vi "1D Look-Up Table.vi"   [LabVIEW 2017, in "NI_AdvCtrl_nonlinear.lvlib"]
doc: "LabVIEW no longer supports this VI. You can obtain similar functionality by installing the LabVIEW Simulation Module.\n\nSearches for an element in a given 1D list that has a fractional index (interpolation)."
uses:
  <vilib>/addons/control/advanced/NI_AdvCtrl_nonlinear.lvlib
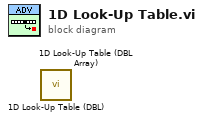
[diagram p0: block diagram]
diagram:
  n1 = call <vilib>:"1D Look-Up Table (DBL).vi"() -> ()  [unwired: 3 in, 1 out]
  n2 = call <vilib>:"1D Look-Up Table (DBL Array).vi"() -> ()  [unwired: 3 in, 1 out]
